vi "test_read-nmea-data2.vi"() -> ()   [LabVIEW 2019] (continued)
,20,06,64,047,26,1*6D\n\t\n15:10:46.40\tF9P\t$GPGSV,3,2,09,09,45,074,19,12,24,277,21,17,33,153,26,19,53,157,25,1*64\n\t\n15:10:46.42\tF9P\t$GPGSV,3,3,09,25,12,307,17,1*5B\n\t\n15:10:46.44\tF9P\t$GPGSV,3,1,09,02,54,318,,04,18,044,,05,37,247,09,06,64,047,15,6*66\n\t\n15:10:46.46\tF9P\t$GPGSV,3,2,09,09,45,074,,12,24,277,,17,33,153,18,19,53,157,,6*62\n\t\n15:10:46.48\tF9P\t$GPGSV,3,3,09,25,12,307,14,6*5F\n\t\n15:10:46.50\tF9P\t$GLGSV,2,1,08,69,12,031,,70,72,041,,71,51,205,19,72,03,209,,1*7A\n\t\n15:10:46.52\tF9P\t$GLGSV,2,2,08,77,01,326,,84,20,122,11,85,70,065,23,86,36,330,,1*7A\n\t\n15:10:46.54\tF9P\t$GLGSV,2,1,08,69,12,031,,70,72,041,,71,51,205,21,72,03,209,,3*73\n\t\n15:10:46.56\tF9P\t$GLGSV,2,2,08,77,01,326,,84,20,122,12,85,70,065,19,86,36,330,,3*72\n\t\n15:10:46.58\tF9P\t$GAGSV,2,1,08,02,09,298,10,04,66,119,25,09,31,193,21,11,71,357,21,7*7C\n\t\n15:10:46.60\tF9P\t$GAGSV,2,2,08,12,40,102,15,19,27,045,15,25,09,249,,36,25,308,14,7*7E\n\t\n15:10:46.62\tF9P\t$GAGSV,2,1,08,02,09,298,,04,66,119,,09,31,193,,11,71,357,,2*7F\n\t\n15:10:46.64\tF9P\t$GAGSV,2,2,08,12,40,102,,19,27,045,,25,09,249,,36,25,308,,2*7E\n\t\n15:10:46.66\tF9P\t$GBGSV,1,1,03,11,50,131,20,14,87,138,20,33,60,219,21,1*4C\n\t\n15:10:46.68\tF9P\t$GBGSV,1,1,03,11,50,131,,14,87,138,,33,60,219,,3*4D\n\t\n15:10:46.70\tF9P\t$GNGLL,3723.55761,N,12656.88740,E,061048.00,A,A*7C\n\t\n15:10:46.72\tF9P\t\t\n15:10:46.74\tF9P\t\t\n15:10:46.76\tF9P\t\t\n15:10:46.78\tF9P\t\t\n15:10:46.80\tF9P\t\t\n15:10:46.82\tF9P\t\t\n15:10:46.84\tF9P\t\t\n15:10:46.86\tF9P\t\t\n15:10:46.88\tF9P\t\t\n15:10:46.90\tF9P\t\t\n15:10:46.92\tF9P\t\t\n15:10:46.94\tF9P\t\t\n15:10:46.96\tF9P\t\t\n15:10:46.98\tF9P\t\t\n15:10:47.00\tF9P\t\t\n15:10:47.02\tF9P\t\t\n15:10:47.04\tF9P\t\t\n15:10:47.06\tF9P\t\t\n15:10:47.08\tF9P\t\t\n15:10:47.10\tF9P\t\t\n15:10:47.12\tF9P\t\t\n15:10:47.14\tF9P\t\t\n15:10:47.16\tF9P\t\t\n15:10:47.18\tF9P\t\t\n15:10:47.20\tF9P\t\t\n15:10:47.22\tF9P\t\t\n15:10:47.24\tF9P\t$GNRMC,061049.00,A,3723.55703,N,12656.88742,E,1.777,,250720,,,A,V*1C\n\t\n15:10:47.26\tF9P\t$GNVTG,,T,,M,1.777,N,3.290,K,A*33\n\t\n15:10:47.28\tF9P\t$GNGGA,061049.00,3723.55703,N,12656.88742,E,1,12,0.64,65.5,M,18.5,M,,*75\n\t\n15:10:47.30\tF9P\t$GNGSA,A,3,12,06,19,05,17,09,04,02,,,,,1.18,0.64,1.00,1*0B\n\t\n15:10:47.32\tF9P\t$GNGSA,A,3,85,71,84,,,,,,,,,,1.18,0.64,1.00,2*0E\n\t\n15:10:47.34\tF9P\t$GNGSA,A,3,36,19,11,04,09,12,,,,,,,1.18,0.64,1.00,3*0B\n\t\n15:10:47.36\tF9P\t$GNGSA,A,3,14,11,33,,,,,,,,,,1.18,0.64,1.00,4*0A\n\t\n15:10:47.38\tF9P\t$GPGSV,3,1,09,02,54,318,33,04,18,044,16,05,37,247,20,06,64,047,26,1*6D\n\t\n15:10:47.40\tF9P\t$GPGSV,3,2,09,09,45,074,17,12,24,277,22,17,33,153,26,19,53,157,24,1*68\n\t\n15:10:47.42\tF9P\t$GPGSV,3,3,09,25,12,307,16,1*5A\n\t\n15:10:47.44\tF9P\t$GPGSV,3,1,09,02,54,318,,04,18,044,,05,37,247,,06,64,047,13,6*69\n\t\n15:10:47.46\tF9P\t$GPGSV,3,2,09,09,45,074,,12,24,277,,17,33,153,17,19,53,157,,6*6D\n\t\n15:10:47.48\tF9P\t$GPGSV,3,3,09,25,12,307,,6*5A\n\t\n15:10:47.50\tF9P\t$GLGSV,2,1,08,69,12,031,,70,72,041,,71,51,205,20,72,03,209,,1*70\n\t\n15:10:47.52\tF9P\t$GLGSV,2,2,08,77,01,326,,84,20,122,09,85,70,065,23,86,36,330,,1*73\n\t\n15:10:47.54\tF9P\t$GLGSV,2,1,08,69,12,031,,70,72,041,,71,51,205,22,72,03,209,,3*70\n\t\n15:10:47.56\tF9P\t$GLGSV,2,2,08,77,01,326,,84,20,122,12,85,70,065,18,86,36,330,,3*73\n\t\n15:10:47.58\tF9P\t$GAGSV,2,1,08,02,09,298,09,04,66,119,23,09,31,193,20,11,71,357,21,7*73\n\t\n15:10:47.60\tF9P\t$GAGSV,2,2,08,12,40,102,15,19,27,045,13,25,09,249,,36,25,308,10,7*7C\n\t\n15:10:47.62\tF9P\t$GAGSV,2,1,08,02,09,298,,04,66,119,,09,31,193,,11,71,357,,2*7F\n\t\n15:10:47.64\tF9P\t$GAGSV,2,2,08,12,40,102,,19,27,045,,25,09,249,,36,25,308,,2*7E\n\t\n15:10:47.66\tF9P\t$GBGSV,1,1,03,11,50,131,21,14,87,138,20,33,60,219,21,1*4D\n\t\n15:10:47.68\tF9P\t$GBGSV,1,1,03,11,50,131,26,14,87,138,,33,60,219,,3*49\n\t\n15:10:47.70\tF9P\t$GNGLL,3723.55703,N,12656.88742,E,061049.00,A,A*7B\n\t\n15:10:47.72\tF9P\t\t\n15:10:47.74\tF9P\t\t\n15:10:47.76\tF9P\t\t\n15:10:47.78\tF9P\t\t\n15:10:47.80\tF9P\t\t\n15:10:47.82\tF9P\t\t\n15:10:47.84\tF9P\t\t\n15:10:47.86\tF9P\t\t\n15:10:47.88\tF9P\t\t\n15:10:47.90\tF9P\t\t\n15:10:47.92\tF9P\t\t\n15:10:47.94\tF9P\t\t\n15:10:47.96\tF9P\t\t\n15:10:47.98\tF9P\t\t\n15:10:48.00\tF9P\t\t\n15:10:48.02\tF9P\t\t\n15:10:48.04\tF9P\t\t\n15:10:48.06\tF9P\t\t\n15:10:48.08\tF9P\t\t\n15:10:48.10\tF9P\t\t\n15:10:48.12\tF9P\t\t\n15:10:48.14\tF9P\t\t\n15:10:48.16\tF9P\t\t\n15:10:48.18\tF9P\t\t\n15:10:48.20\tF9P\t\t\n15:10:48.22\tF9P\t\t\n15:10:48.24\tF9P\t$GNRMC,061050.00,A,3723.55644,N,12656.88759,E,2.146,158.95,250720,,,A,V*05\n\t\n15:10:48.26\tF9P\t$GNVTG,158.95,T,,M,2.146,N,3.975,K,A*2A\n\t\n15:10:48.28\tF9P\t$GNGGA,061050.00,3723.55644,N,12656.88759,E,1,12,0.64,65.9,M,18.5,M,,*79\n\t\n15:10:48.30\tF9P\t$GNGSA,A,3,12,06,19,05,17,09,04,02,,,,,1.18,0.64,1.00,1*0B\n\t\n15:10:48.32\tF9P\t$GNGSA,A,3,85,71,84,,,,,,,,,,1.18,0.64,1.00,2*0E\n\t\n15:10:48.34\tF9P\t$GNGSA,A,3,36,19,11,04,09,12,,,,,,,1.18,0.64,1.00,3*0B\n\t\n15:10:48.36\tF9P\t$GNGSA,A,3,14,11,33,,,,,,,,,,1.18,0.64,1.00,4*0A\n\t\n15:10:48.38\tF9P\t$GPGSV,3,1,09,02,54,318,33,04,18,044,14,05,37,247,21,06,64,047,35,1*6C\n\t\n15:10:48.40\tF9P\t$GPGSV,3,2,09,09,45,074,18,12,24,277,24,17,33,153,26,19,53,157,24,1*61\n\t\n15:10:48.42\tF9P\t$GPGSV,3,3,09,25,12,307,17,1*5B\n\t\n15:10:48.44\tF9P\t$GPGSV,3,1,09,02,54,318,,04,18,044,,05,37,247,,06,64,047,14,6*6E\n\t\n15:10:48.46\tF9P\t$GPGSV,3,2,09,09,45,074,,12,24,277,,17,33,153,17,19,53,157,,6*6D\n\t\n15:10:48.48\tF9P\t$GPGSV,3,3,09,25,12,307,,6*5A\n\t\n15:10:48.50\tF9P\t$GLGSV,2,1,08,69,12,031,,70,72,041,,71,51,205,20,72,03,209,,1*70\n\t\n15:10:48.52\tF9P\t$GLGSV,2,2,08,77,01,326,,84,20,122,09,85,70,065,21,86,36,330,,1*71\n\t\n15:10:48.54\tF9P\t$GLGSV,2,1,08,69,12,031,,70,72,041,,71,51,205,21,72,03,209,,3*73\n\t\n15:10:48.56\tF9P\t$GLGSV,2,2,08,77,01,326,,84,20,122,10,85,70,065,19,86,36,330,,3*70\n\t\n15:10:48.58\tF9P\t$GAGSV,2,1,08,02,09,298,10,04,66,119,24,09,31,193,20,11,71,357,20,7*7D\n\t\n15:10:48.60\tF9P\t$GAGSV,2,2,08,12,40,102,16,19,27,045,12,25,09,249,,36,25,308,13,7*7D\n\t\n15:10:48.62\tF9P\t$GAGSV,2,1,08,02,09,298,,04,66,119,,09,31,193,,11,71,357,,2*7F\n\t\n15:10:48.64\tF9P\t$GAGSV,2,2,08,12,40,102,,19,27,045,,25,09,249,,36,25,308,,2*7E\n\t\n15:10:48.66\tF9P\t$GBGSV,1,1,03,11,50,131,20,14,87,138,21,33,60,219,21,1*4D\n\t\n15:10:48.68\tF9P\t$GBGSV,1,1,03,11,50,131,32,14,87,138,,33,60,219,,3*4C\n\t\n15:10:48.70\tF9P\t$GNGLL,3723.55644,N,12656.88759,E,061050.00,A,A*7B\n\t\n15:10:48.72\tF9P\t\t\n15:10:48.74\tF9P\t\t\n15:10:48.76\tF9P\t\t\n15:10:48.78\tF9P\t\t\n15:10:48.80\tF9P\t\t\n15:10:48.82\tF9P\t\t\n15:10:48.84\tF9P\t\t\n15:10:48.86\tF9P\t\t\n15:10:48.88\tF9P\t\t\n15:10:48.90\tF9P\t\t\n15:10:48.92\tF9P\t\t\n15:10:48.94\tF9P\t\t\n15:10:48.96\tF9P\t\t\n15:10:48.98\tF9P\t\t\n15:10:49.00\tF9P\t\t\n15:10:49.02\tF9P\t\t\n15:10:49.04\tF9P\t\t\n15:10:49.06\tF9P\t\t\n15:10:49.08\tF9P\t\t\n15:10:49.10\tF9P\t\t\n15:10:49.12\tF9P\t\t\n15:10:49.14\tF9P\t\t\n15:10:49.16\tF9P\t\t\n15:10:49.18\tF9P\t\t\n15:10:49.20\tF9P\t\t\n15:10:49.22\tF9P\t\t\n15:10:49.24\tF9P\t$GNRMC,061051.00,A,3723.55587,N,12656.88770,E,2.092,,250720,,,A,V*15\n\t\n15:10:49.26\tF9P\t$GNVTG,,T,,M,2.092,N,3.874,K,A*3C\n\t\n15:10:49.28\tF9P\t$GNGGA,061051.00,3723.55587,N,12656.88770,E,1,12,0.67,66.1,M,18.5,M,,*77\n\t\n15:10:49.30\tF9P\t$GNGSA,A,3,12,06,19,05,17,09,04,02,,,,,1.23,0.67,1.03,1*03\n\t\n15:10:49.32\tF9P\t$GNGSA,A,3,85,71,84,,,,,,,,,,1.23,0.67,1.03,2*06\n\t\n15:10:49.34\tF9P\t$GNGSA,A,3,36,11,04,09,12,,,,,,,,1.23,0.67,1.03,3*0B\n\t\n15:10:49.36\tF9P\t$GNGSA,A,3,14,11,33,,,,,,,,,,1.23,0.67,1.03,4*02\n\t\n15:10:49.38\tF9P\t$GPGSV,3,1,09,02,54,318,34,04,18,044,13,05,37,247,21,06,64,047,26,1*6E\n\t\n15:10:49.40\tF9P\t$GPGSV,3,2,09,09,45,074,17,12,24,277,21,17,33,153,24,19,53,157,23,1*6E\n\t\n15:10:49.42\tF9P\t$GPGSV,3,3,09,25,12,307,20,1*5F\n\t\n15:10:49.44\tF9P\t$GPGSV,3,1,09,02,54,318,,04,18,044,,05,37,247,,06,64,047,15,6*6F\n\t\n15:10:49.46\tF9P\t$GPGSV,3,2,09,09,45,074,,12,24,277,,17,33,153,16,19,53,157,,6*6C\n\t\n15:10:49.48\tF9P\t$GPGSV,3,3,09,25,12,307,,6*5A\n\t\n15:10:49.50\tF9P\t$GLGSV,2,1,08,69,12,031,,70,72,041,,71,51,205,19,72,03,209,,1*7A\n\t\n15:10:49.52\tF9P\t$GLGSV,2,2,08,77,01,326,,84,20,122,10,85,70,065,19,86,36,330,,1*72\n\t\n15:10:49.54\tF9P\t$GLGSV,2,1,08,69,12,031,,70,72,041,,71,51,205,22,72,03,209,,3*70\n\t\n15:10:49.56\tF9P\t$GLGSV,2,2,08,77,01,326,,84,20,122,18,85,70,065,19,86,36,330,,3*78\n\t\n15:10:49.58\tF9P\t$GAGSV,2,1,08,02,09,298,08,04,66,119,24,09,31,193,19,11,71,357,20,7*7E\n\t\n15:10:49.60\tF9P\t$GAGSV,2,2,08,12,40,102,15,19,27,045,09,25,09,249,,36,25,308,10,7*77\n\t\n15:10:49.62\tF9P\t$GAGSV,2,1,08,02,09,298,,04,66,119,,09,31,193,,11,71,357,,2*7F\n\t\n15:10:49.64\tF9P\t$GAGSV,2,2,08,12,40,102,,19,27,045,,25,09,249,,36,25,308,,2*7E\n\t\n15:10:49.66\tF9P\t$GBGSV,1,1,03,11,50,131,18,14,87,138,21,33,60,219,22,1*45\n\t\n15:10:49.68\tF9P\t$GBGSV,1,1,03,11,50,131,27,14,87,138,,33,60,219,,3*48\n\t\n15:10:49.70\tF9P\t$GNGLL,3723.55587,N,12656.88770,E,061051.00,A,A*7D\n\t\n15:10:49.72\tF9P\t\t\n15:10:49.74\tF9P\t\t\n15:10:49.76\tF9P\t\t\n15:10:49.78\tF9P\t\t\n15:10:49.80\tF9P\t\t\n15:10:49.82\tF9P\t\t\n15:10:49.84\tF9P\t\t\n15:10:49.86\tF9P\t\t\n15:10:49.88\tF9P\t\t\n15:10:49.90\tF9P\t\t\n15:10:49.92\tF9P\t\t\n15:10:49.94\tF9P\t\t\n15:10:49.96\tF9P\t\t\n15:10:49.98\tF9P\t\t\n15:10:50.00\tF9P\t\t\n15:10:50.02\tF9P\t\t\n15:10:50.04\tF9P\t\t\n15:10:50.06\tF9P\t\t\n15:10:50.08\tF9P\t\t\n15:10:50.10\tF9P\t\t\n15:10:50.12\tF9P\t\t\n15:10:50.14\tF9P\t\t\n15:10:50.16\tF9P\t\t\n15:10:50.18\tF9P\t\t\n15:10:50.20\tF9P\t\t\n15:10:50.22\tF9P\t\t\n15:10:50.24\tF9P\t$GNRMC,061052.00,A,3723.55538,N,12656.88805,E,1.856,,250720,,,A,V*1C\n\t\n15:10:50.26\tF9P\t$GNVTG,,T,,M,1.856,N,3.438,K,A*3B\n\t\n15:10:50.28\tF9P\t$GNGGA,061052.00,3723.55538,N,12656.88805,E,1,12,0.64,66.1,M,18.5,M,,*7E\n\t\n15:10:50.30\tF9P\t$GNGSA,A,3,12,06,19,05,17,09,04,02,,,,,1.18,0.64,1.00,1*0B\n\t\n15:10:50.32\tF9P\t$GNGSA,A,3,85,71,84,,,,,,,,,,1.18,0.64,1.00,2*0E\n\t\n15:10:50.34\tF9P\t$GNGSA,A,3,36,19,11,04,09,12,,,,,,,1.18,0.64,1.00,3*0B\n\t\n15:10:50.36\tF9P\t$GNGSA,A,3,14,11,33,,,,,,,,,,1.18,0.64,1.00,4*0A\n\t\n15:10:50.38\tF9P\t$GPGSV,3,1,09,02,54,318,34,04,18,044,14,05,37,247,21,06,64,047,32,1*6C\n\t\n15:10:50.40\tF9P\t$GPGSV,3,2,09,09,45,074,16,12,24,277,21,17,33,153,22,19,53,157,22,1*68\n\t\n15:10:50.42\tF9P\t$GPGSV,3,3,09,25,12,307,21,1*5E\n\t\n15:10:50.44\tF9P\t$GPGSV,3,1,09,02,54,318,,04,18,044,,05,37,247,,06,64,047,15,6*6F\n\t\n15:10:50.46\tF9P\t$GPGSV,3,2,09,09,45,074,,12,24,277,,17,33,153,14,19,53,157,,6*6E\n\t\n15:10:50.48\tF9P\t$GPGSV,3,3,09,25,12,307,,6*5A\n\t\n15:10:50.50\tF9P\t$GLGSV,2,1,08,69,12,031,,70,72,041,,71,51,205,18,72,03,209,,1*7B\n\t\n15:10:50.52\tF9P\t$GLGSV,2,2,08,77,01,326,,84,20,122,11,85,70,065,19,86,36,330,,1*73\n\t\n15:10:50.54\tF9P\t$GLGSV,2,1,08,69,12,031,,70,72,041,,71,51,205,23,72,03,209,,3*71\n\t\n15:10:50.56\tF9P\t$GLGSV,2,2,08,77,01,326,,84,20,122,14,85,70,065,18,86,36,330,,3*75\n\t\n15:10:50.58\tF9P\t$GAGSV,2,1,08,02,09,298,09,04,66,119,24,09,31,193,19,11,71,357,21,7*7E\n\t\n15:10:50.60\tF9P\t$GAGSV,2,2,08,12,40,102,17,19,27,045,10,25,09,249,,36,25,308,13,7*7E\n\t\n15:10:50.62\tF9P\t$GAGSV,2,1,08,02,09,298,,04,66,119,,09,31,193,,11,71,357,,2*7F\n\t\n15:10:50.64\tF9P\t$GAGSV,2,2,08,12,40,102,26,19,27,045,,25,09,249,,36,25,308,,2*7A\n\t\n15:10:50.66\tF9P\t$GBGSV,1,1,03,11,50,131,19,14,87,138,20,33,60,219,20,1*47\n\t\n15:10:50.68\tF9P\t$GBGSV,1,1,03,11,50,131,29,14,87,138,,33,60,219,,3*46\n\t\n15:10:50.70\tF9P\t$GNGLL,3723.55538,N,12656.88805,E,061052.00,A,A*77\n\t\n15:10:50.72\tF9P\t\t\n15:10:50.74\tF9P\t\t\n15:10:50.76\tF9P\t\t\n15:10:50.78\tF9P\t\t\n15:10:50.80\tF9P\t\t\n15:10:50.82\tF9P\t\t\n15:10:50.84\tF9P\t\t\n15:10:50.86\tF9P\t\t\n15:10:50.88\tF9P\t\t\n15:10:50.90\tF9P\t\t\n15:10:50.92\tF9P\t\t\n15:10:50.94\tF9P\t\t\n15:10:50.96\tF9P\t\t\n15:10:50.98\tF9P\t\t\n15:10:51.00\tF9P\t\t\n15:10:51.02\tF9P\t\t\n15:10:51.04\tF9P\t\t\n15:10:51.06\tF9P\t\t\n15:10:51.08\tF9P\t\t\n15:10:51.10\tF9P\t\t\n15:10:51.12\tF9P\t\t\n15:10:51.14\tF9P\t\t\n15:10:51.16\tF9P\t\t\n15:10:51.18\tF9P\t\t\n15:10:51.20\tF9P\t\t\n15:10:51.22\tF9P\t\t\n15:10:51.24\tF9P\t$GNRMC,061053.00,A,3723.55490,N,12656.88844,E,1.738,,250720,,,A,V*1C\n\t\n15:10:51.26\tF9P\t$GNVTG,,T,,M,1.738,N,3.218,K,A*38\n\t\n15:10:51.28\tF9P\t$GNGGA,061053.00,3723.55490,N,12656.88844,E,1,12,0.64,66.3,M,18.5,M,,*7B\n\t\n15:10:51.30\tF9P\t$GNGSA,A,3,12,06,19,05,17,09,04,02,,,,,1.18,0.64,0.99,1*0A\n\t\n15:10:51.32\tF9P\t$GNGSA,A,3,85,71,84,,,,,,,,,,1.18,0.64,0.99,2*0F\n\t\n15:10:51.34\tF9P\t$GNGSA,A,3,36,19,11,04,09,12,,,,,,,1.18,0.64,0.99,3*0A\n\t\n15:10:51.36\tF9P\t$GNGSA,A,3,14,11,33,,,,,,,,,,1.18,0.64,0.99,4*0B\n\t\n15:10:51.38\tF9P\t$GPGSV,3,1,09,02,54,318,29,04,18,044,14,05,37,247,22,06,64,047,33,1*62\n\t\n15:10:51.40\tF9P\t$GPGSV,3,2,09,09,45,074,16,12,24,277,21,17,33,153,23,19,53,157,23,1*68\n\t\n15:10:51.42\tF9P\t$GPGSV,3,3,09,25,12,307,20,1*5F\n\t\n15:10:51.44\tF9P\t$GPGSV,3,1,09,02,54,318,,04,18,044,,05,37,247,,06,64,047,15,6*6F\n\t\n15:10:51.46\tF9P\t$GPGSV,3,2,09,09,45,074,,12,24,277,,17,33,153,13,19,53,157,,6*69\n\t\n15:10:51.48\tF9P\t$GPGSV,3,3,09,25,12,307,,6*5A\n\t\n15:10:51.50\tF9P\t$GLGSV,2,1,08,69,12,031,,70,72,041,,71,51,205,17,72,03,209,,1*74\n\t\n15:10:51.52\tF9P\t$GLGSV,2,2,08,77,01,326,,84,20,122,11,85,70,065,28,86,36,330,,1*71\n\t\n15:10:51.54\tF9P\t$GLGSV,2,1,08,69,12,031,,70,72,041,,71,51,205,22,72,03,209,,3*70\n\t\n15:10:51.56\tF9P\t$GLGSV,2,2,08,77,01,326,,84,20,122,16,85,70,065,19,86,36,330,,3*76\n\t\n15:10:51.58\tF9P\t$GAGSV,2,1,08,02,09,298,08,04,66,119,31,09,31,193,20,11,71,357,21,7*71\n\t\n15:10:51.60\tF9P\t$GAGSV,2,2,08,12,40,102,19,19,27,045,10,25,09,249,,36,25,308,13,7*70\n\t\n15:10:51.62\tF9P\t$GAGSV,2,1,08,02,09,298,,04,66,119,,09,31,193,,11,71,357,,2*7F\n\t\n15:10:51.64\tF9P\t$GAGSV,2,2,08,12,40,102,24,19,27,045,,25,09,249,,36,25,308,,2*78\n\t\n15:10:51.66\tF9P\t$GBGSV,1,1,03,11,50,131,22,14,87,138,20,33,60,219,21,1*4E\n\t\n15:10:51.68\tF9P\t$GBGSV,1,1,03,11,50,131,32,14,87,138,,33,60,219,,3*4C\n\t\n15:10:51.70\tF9P\t$GNGLL,3723.55490,N,12656.88844,E,061053.00,A,A*70\n\t\n15:10:51.72\tF9P\t\t\n15:10:51.74\tF9P\t\t\n15:10:51.76\tF9P\t\t\n15:10:51.78\tF9P\t\t\n15:10:51.80\tF9P\t\t\n15:10:51.82\tF9P\t\t\n15:10:51.84\tF9P\t\t\n15:10:51.86\tF9P\t\t\n15:10:51.88\tF9P\t\t\n15:10:51.90\tF9P\t\t\n15:10:51.92\tF9P\t\t\n15:10:51.94\tF9P\t\t\n15:10:51.96\tF9P\t\t\n15:10:51.98\tF9P\t\t\n15:10:52.00\tF9P\t\t\n15:10:52.02\tF9P\t\t\n15:10:52.04\tF9P\t\t\n15:10:52.06\tF9P\t\t\n15:10:52.08\tF9P\t\t\n15:10:52.10\tF9P\t\t\n15:10:52.12\tF9P\t\t\n15:10:52.14\tF9P\t\t\n15:10:52.16\tF9P\t\t\n15:10:52.18\tF9P\t\t\n15:10:52.20\tF9P\t\t\n15:10:52.22\tF9P\t\t\n15:10:52.24\tF9P\t$GNRMC,061054.00,A,3723.55439,N,12656.88882,E,1.892,,250720,,,A,V*1D\n\t\n15:10:52.26\tF9P\t$GNVTG,,T,,M,1.892,N,3.505,K,A*3C\n\t\n15:10:52.28\tF9P\t$GNGGA,061054.00,3723.55439,N,12656.88882,E,1,12,0.64,66.4,M,18.5,M,,*72\n\t\n15:10:52.30\tF9P\t$GNGSA,A,3,12,06,19,05,17,09,04,02,,,,,1.18,0.64,0.99,1*0A\n\t\n15:10:52.32\tF9P\t$GNGSA,A,3,85,71,84,,,,,,,,,,1.18,0.64,0.99,2*0F\n\t\n15:10:52.34\tF9P\t$GNGSA,A,3,36,19,11,04,09,12,,,,,,,1.18,0.64,0.99,3*0A\n\t\n15:10:52.36\tF9P\t$GNGSA,A,3,14,11,33,,,,,,,,,,1.18,0.64,0.99,4*0B\n\t\n15:10:52.38\tF9P\t$GPGSV,3,1,09,02,54,318,30,04,18,044,15,05,37,247,24,06,64,047,27,1*68\n\t\n15:10:52.40\tF9P\t$GPGSV,3,2,09,09,45,074,17,12,24,277,23,17,33,153,24,19,53,157,23,1*6C\n\t\n15:10:52.42\tF9P\t$GPGSV,3,3,09,25,12,307,19,1*55\n\t\n15:10:52.44\tF9P\t$GPGSV,3,1,09,02,54,318,,04,18,044,,05,37,247,,06,64,047,15,6*6F\n\t\n15:10:52.46\tF9P\t$GPGSV,3,2,09,09,45,074,,12,24,277,,17,33,153,13,19,53,157,,6*69\n\t\n15:10:52.48\tF9P\t$GPGSV,3,3,09,25,12,307,,6*5A\n\t\n15:10:52.50\tF9P\t$GLGSV,2,1,08,69,12,031,,70,72,041,,71,51,205,17,72,03,209,,1*74\n\t\n15:10:52.52\tF9P\t$GLGSV,2,2,08,77,01,326,,84,20,122,11,85,70,065,26,86,36,330,,1*7F\n\t\n15:10:52.54\tF9P\t$GLGSV,2,1,08,69,12,031,,70,72,041,,71,51,205,24,72,03,209,,3*76\n\t\n15:10:52.56\tF9P\t$GLGSV,2,2,08,77,01,326,,84,20,122,15,85,70,065,19,86,36,330,,3*75\n\t\n15:10:52.58\tF9P\t$GAGSV,2,1,08,02,09,298,09,04,66,119,25,09,31,193,21,11,71,357,21,7*74\n\t\n15:10:52.60\tF9P\t$GAGSV,2,2,08,12,40,102,20,19,27,045,09,25,09,249,,36,25,308,12,7*73\n\t\n15:10:52.62\tF9P\t$GAGSV,2,1,08,02,09,298,,04,66,119,,09,31,193,,11,71,357,,2*7F\n\t\n15:10:52.64\tF9P\t$GAGSV,2,2,08,12,40,102,21,19,27,045,,25,09,249,,36,25,308,,2*7D\n\t\n15:10:52.66\tF9P\t$GBGSV,1,1,03,11,50,131,23,14,87,138,22,33,60,219,21,1*4D\n\t\n15:10:52.68\tF9P\t$GBGSV,1,1,03,11,50,131,,14,87,138,,33,60,219,,3*4D\n\t\n15:10:52.70\tF9P\t$GNGLL,3723.55439,N,12656.88882,E,061054.00,A,A*7E\n\t\n15:10:52.72\tF9P\t\t\n15:10:52.74\tF9P\t\t\n15:10:52.76\tF9P\t\t\n15:10:52.78\tF9P\t\t\n15:10:52.80\tF9P\t\t\n15:10:52.82\tF9P\t\t\n15:10:52.84\tF9P\t\t\n15:10:52.86\tF9P\t\t\n15:10:52.88\tF9P\t\t\n15:10:52.90\tF9P\t\t\n15:10:52.92\tF9P\t\t\n15:10:52.94\tF9P\t\t\n15:10:52.96\tF9P\t\t\n15:10:52.98\tF9P\t\t\n15:10:53.00\tF9P\t\t\n15:10:53.02\tF9P\t\t\n15:10:53.04\tF9P\t\t\n15:10:53.06\tF9P\t\t\n15:10:53.08\tF9P\t\t\n15:10:53.10\tF9P\t\t\n15:10:53.12\tF9P\t\t\n15:10:53.14\tF9P\t\t\n15:10:53.16\tF9P\t\t\n15:10:53.18\tF9P\t\t\n15:10:53.20\tF9P\t\t\n15:10:53.22\tF9P\t\t\n15:10:53.24\tF9P\t$GNRMC,061055.00,A,3723.55366,N,12656.88903,E,2.416,160.42,250720,,,A,V*05\n\t\n15:10:53.26\tF9P\t$GNVTG,160.42,T,,M,2.416,N,4.475,K,A*21\n\t\n15:10:53.28\tF9P\t$GNGGA,061055.00,3723.55366,N,12656.88903,E,1,12,0.64,67.0,M,18.5,M,,*73\n\t\n15:10:53.30\tF9P\t$GNGSA,A,3,12,06,19,05,17,09,04,02,,,,,1.18,0.64,0.99,1*0A\n\t\n15:10:53.32\tF9P\t$GNGSA,A,3,85,71,84,,,,,,,,,,1.18,0.64,0.99,2*0F\n\t\n15:10:53.34\tF9P\t$GNGSA,A,3,36,19,11,04,09,12,,,,,,,1.18,0.64,0.99,3*0A\n\t\n15:10:53.36\tF9P\t$GNGSA,A,3,14,11,33,,,,,,,,,,1.18,0.64,0.99,4*0B\n\t\n15:10:53.38\tF9P\t$GPGSV,3,1,09,02,54,318,30,04,18,044,13,05,37,247,23,06,64,047,28,1*66\n\t\n15:10:53.40\tF9P\t$GPGSV,3,2,09,09,45,074,18,12,24,277,25,17,33,153,25,19,53,157,24,1*63\n\t\n15:10:53.42\tF9P\t$GPGSV,3,3,09,25,12,307,17,1*5B\n\t\n15:10:53.44\tF9P\t$GPGSV,3,1,09,02,54,318,,04,18,044,,05,37,247,,06,64,047,17,6*6D\n\t\n15:10:53.46\tF9P\t$GPGSV,3,2,09,09,45,074,,12,24,277,,17,33,153,13,19,53,157,,6*69\n\t\n15:10:53.48\tF9P\t$GPGSV,3,3,09,25,12,307,,6*5A\n\t\n15:10:53.50\tF9P\t$GLGSV,2,1,08,69,12,031,,70,72,041,,71,51,205,16,72,03,209,,1*75\n\t\n15:10:53.52\tF9P\t$GLGSV,2,2,08,77,01,326,,84,20,122,10,85,70,065,25,86,36,330,,1*7D\n\t\n15:10:53.54\tF9P\t$GLGSV,2,1,08,69,12,031,,70,72,041,,71,51,205,23,72,03,209,,3*71\n\t\n15:10:53.56\tF9P\t$GLGSV,2,2,08,77,01,326,,84,20,122,15,85,70,065,20,86,36,330,,3*7F\n\t\n15:10:53.58\tF9P\t$GAGSV,2,1,08,02,09,298,11,04,66,119,25,09,31,193,21,11,71,357,19,7*76\n\t\n15:10:53.60\tF9P\t$GAGSV,2,2,08,12,40,102,20,19,27,045,08,25,09,249,,36,25,308,10,7*70\n\t\n15:10:53.62\tF9P\t$GAGSV,2,1,08,02,09,298,,04,66,119,27,09,31,193,,11,71,357,,2*7A\n\t\n15:10:53.64\tF9P\t$GAGSV,2,2,08,12,40,102,21,19,27,045,,25,09,249,,36,25,308,,2*7D\n\t\n15:10:53.66\tF9P\t$GBGSV,1,1,03,11,50,131,22,14,87,138,22,33,60,219,21,1*4C\n\t\n15:10:53.68\tF9P\t$GBGSV,1,1,03,11,50,131,35,14,87,138,,33,60,219,,3*4B\n\t\n15:10:53.70\tF9P\t$GNGLL,3723.55366,N,12656.88903,E,061055.00,A,A*7A\n\t\n15:10:53.72\tF9P\t\t\n15:10:53.74\tF9P\t\t\n15:10:53.76\tF9P\t\t\n15:10:53.78\tF9P\t\t\n15:10:53.80\tF9P\t\t\n15:10:53.82\tF9P\t\t\n15:10:53.84\tF9P\t\t\n15:10:53.86\tF9P\t\t\n15:10:53.88\tF9P\t\t\n15:10:53.90\tF9P\t\t\n15:10:53.92\tF9P\t\t\n15:10:53.94\tF9P\t\t\n15:10:53.96\tF9P\t\t\n15:10:53.98\tF9P\t\t\n15:10:54.00\tF9P\t\t\n15:10:54.02\tF9P\t\t\n15:10:54.04\tF9P\t\t\n15:10:54.06\tF9P\t\t\n15:10:54.08\tF9P\t\t\n15:10:54.10\tF9P\t\t\n15:10:54.12\tF9P\t\t\n15:10:54.14\tF9P\t\t\n15:10:54.16\tF9P\t\t\n15:10:54.18\tF9P\t\t\n15:10:54.20\tF9P\t\t\n15:10:54.22\tF9P\t\t\n15:10:54.24\tF9P\t$GNRMC,061056.00,A,3723.55311,N,12656.88974,E,2.196,,250720,,,A,V*14\n\t\n15:10:54.26\tF9P\t$GNVTG,,T,,M,2.196,N,4.067,K,A*34\n\t\n15:10:54.28\tF9P\t$GNGGA,061056.00,3723.55311,N,12656.88974,E,1,12,0.64,66.5,M,18.5,M,,*74\n\t\n15:10:54.30\tF9P\t$GNGSA,A,
